vi "2D array remove invalid numbers.vi"(0 "iteration number\n(when interpolate)":i32, 1 "interpolate":bool, 2 "transpose":bool, 4 "all columns":bool=TRUE, 5 "invalid numbers list":dbl[](array[numeric])=[inf, -inf, 0.0], 6 "min":dbl=-inf, 7 "max":dbl=inf, 8 "menu":T1(ring), 9 "selected coulumn":i32, 10 "array in":dbl[][](array[numeric])=[[2.9e-06, 1031.066], [0.3000111, 1030.889], [0.6000026, 1030.51], [0.9000013, 1029.772], [1.199967, 1028.994], [1.499969, 1028.095], [1.7999, 1027.132], [2.099874, 1026.203], [2.399872, 1025.28], [2.699817, 1024.361], [2.999824, 1023.485], [3.299903, 1022.622], [3.599948, 1021.759], [3.899851, 1020.978], [4.199977, 1020.139], [4.499946, 1019.425], [4.799844, 1018.635], [5.099932, 1017.888], [5.400068, 1017.252], [5.699985, 1016.525], [5.99992, 1015.822], [6.299928, 1015.166], [6.600165, 1014.52], [6.900076, 1013.781], [7.200036, 1013.158], [7.500067, 1012.494], [7.800045, 1011.846], [8.099933, 1011.217], [8.400136, 1010.525], [8.699943, 1009.959], [9.000045, 1009.171], [9.000007, 1009.165], [0.0, 0.0], [0.0, 0.0], [0.0, 0.0], [0.0, 0.0], [0.0, 0.0], [0.0, 0.0], [0.0, 0.0], [0.0, 0.0], [0.0, 0.0], [0.0, 0.0], [0.0, 0.0], [0.0, 0.0], [0.0, 0.0], [0.0, 0.0]]) -> (3 "array out":dbl[][](array[numeric])=[[2.9e-06, 1031.066], [0.3000111, 1030.889], [0.6000026, 1030.51], [0.9000013, 1029.772], [1.199967, 1028.994], [1.499969, 1028.095], [1.7999, 1027.132], [2.099874, 1026.203], [2.399872, 1025.28], [2.699817, 1024.361], [2.999824, 1023.485], [3.299903, 1022.622], [3.599948, 1021.759], [3.899851, 1020.978], [4.199977, 1020.139], [4.499946, 1019.425], [4.799844, 1018.635], [5.099932, 1017.888], [5.400068, 1017.252], [5.699985, 1016.525], [5.99992, 1015.822], [6.299928, 1015.166], [6.600165, 1014.52], [6.900076, 1013.781], [7.200036, 1013.158], [7.500067, 1012.494], [7.800045, 1011.846], [8.099933, 1011.217], [8.400136, 1010.525], [8.699943, 1009.959], [9.000045, 1009.171], [9.000007, 1009.165], [0.0, 0.0], [0.0, 0.0], [0.0, 0.0], [0.0, 0.0], [0.0, 0.0], [0.0, 0.0], [0.0, 0.0], [0.0, 0.0], [0.0, 0.0], [0.0, 0.0], [0.0, 0.0], [0.0, 0.0], [0.0, 0.0], [0.0, 0.0]])   [LabVIEW 2025]
panel:
  # "NaN: not a number"
  # "Filter out the numbers (3 modes) for the whole or slected columns. The filtered numbers\nare removed or replaced by (sinlge or multiple times) interpolated numbers. \nWhen the numbers are to removed the rows containing the numbers are removed too.  \n\n1. Remove numbers in the list and NaN\n2. Remove numbers in the boundary\n3. Remove numbers out of the boundary\n\nFor modes 2 and 3, the default \"min\" and \"max\" numbers are -Inf and +Inf, respectively.\nIf those numbers are not wired, the operation will be done accordingly."
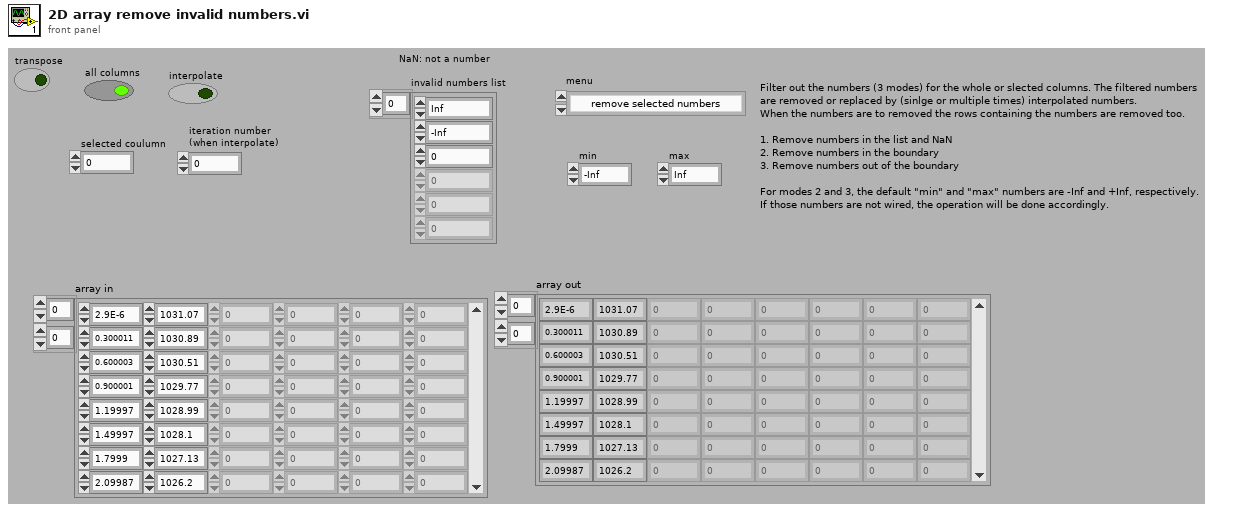
[diagram p1: front panel]
types:
  T1 = enum16{"remove selected numbers", "remove numbers within the range", "remove number out of the range", "no filtering"}
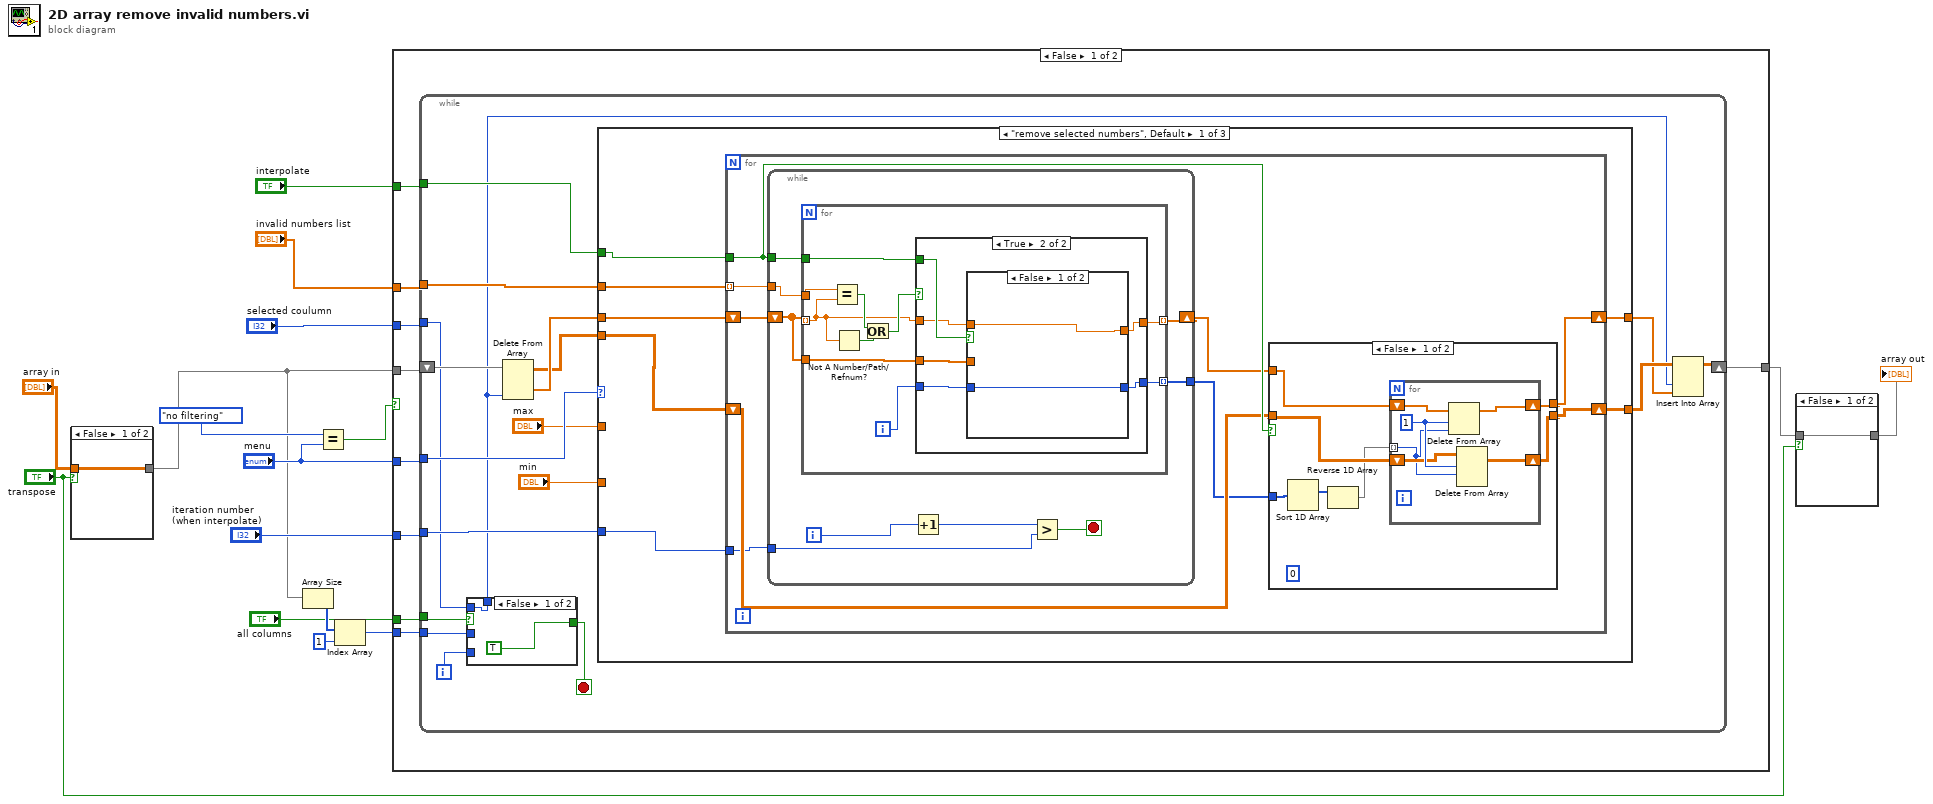
[diagram p0: block diagram]
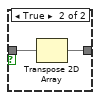
[diagram p2: hidden frame]
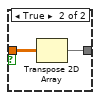
[diagram p3: hidden frame]
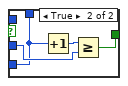
[diagram p4: hidden frame]
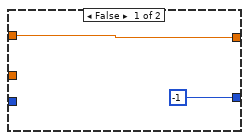
[diagram p5: hidden frame]
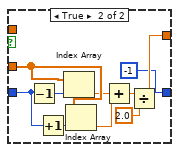
[diagram p6: hidden frame]
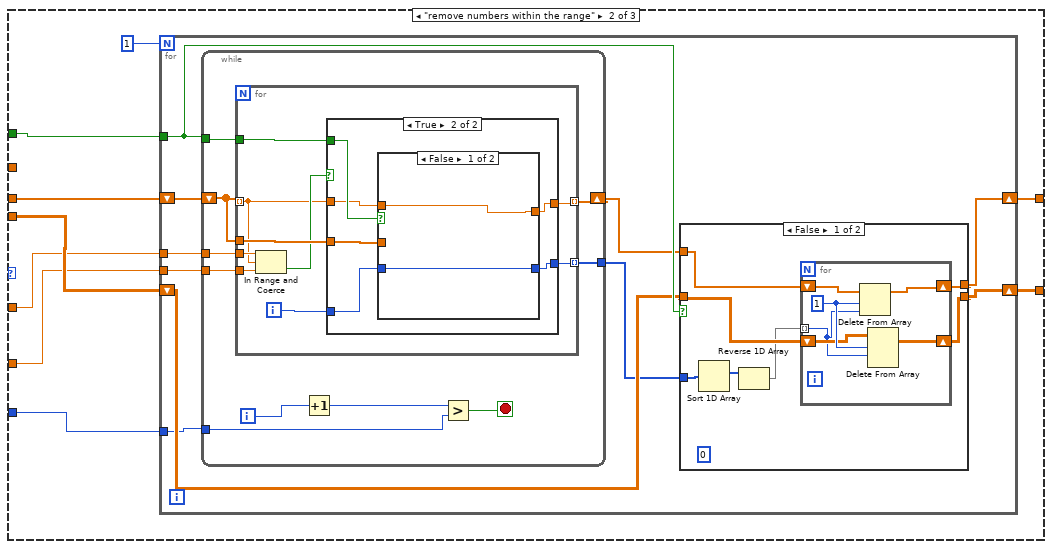
[diagram p8: hidden frame]
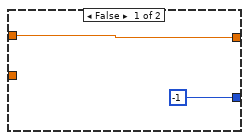
[diagram p9: hidden frame]
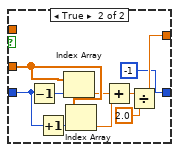
[diagram p10: hidden frame]
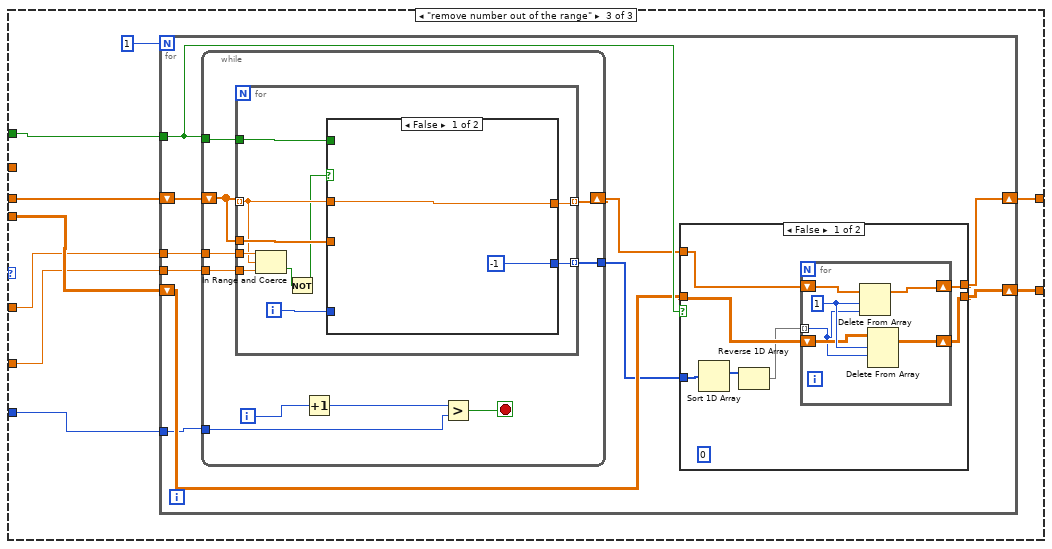
[diagram p12: hidden frame]
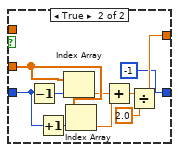
[diagram p14: hidden frame]
diagram:
  n1 = case shown="False" "transpose" {
    tunnel: "array in" -> [w17 w19]
    tunnel: [w17 w18] -> w4
    frame False {
    }
    frame True {
      n2 = Transpose 2D Array(2D array=w19) -> (transposed array=w18:dbl[][])
    }
  }
  n3 = Array Size(array=w4) -> (size(s)=w12:i32[])
  n4 = Equal?(x=T1."no filtering" ("menu"), y="menu") -> (x = y?=w7:bool)
  n5 = Index Array(array=w12, index=1) -> (element=w11:i32)
  n6 = case shown="False" w7 {
    tunnel: "interpolate" -> [w28 _]
    tunnel: "iteration number\n(when interpolate)" -> [w27 _]
    tunnel: "invalid numbers list" -> [w26 _]
    tunnel: "menu" -> [w25 _]
    tunnel: "selected coulumn" -> [w24 _]
    tunnel: w4 -> [w23 w270]
    tunnel: w11 -> [w22 _]
    tunnel: "all columns" -> [w21 _]
    tunnel: [w20 w270] -> w3
    frame False {
      n7 = while {
        tunnel: w28 -> [w46]
        tunnel: w27 -> [w42]
        tunnel: w25 -> [w40]
        shift-right: [w31] -> w20
        shift-left: w23 -> [w45]
        tunnel: w24 -> [w38]
        tunnel: w22 -> [w36]
        tunnel: w21 -> [w35]
        tunnel: w26 -> [w41]
        i -> [w37]
        stop <- w39 stop-if-true
        n8 = case shown="False" w35 {
          tunnel: [TRUE w49] -> w39
          tunnel: [w47 w51] -> w32
          tunnel: w38 -> [w47 _]
          tunnel: w37 -> [_ w51]
          tunnel: w36 -> [_ w52]
          frame False {
          }
          frame True {
            n9 = Increment(x=w51) -> (x+1=w50:i32)
            n10 = Greater Or Equal?(x=w50, y=w52) -> (x >= y?=w49:bool)
          }
        }
        n11 = Delete From Array(array=w45, index (col)=w32) -> (deleted portion=w44:dbl[], array with subset deleted=w43:dbl[][])  [unwired: 2 in]
        n12 = case shown="\"remove selected numbers\", Default" w40 {
          tunnel: w44 -> [w59 w131 w204]
          tunnel: w46 -> [w58 w130 w203]
          tunnel: [w57 w129 w202] -> w34
          tunnel: [w56 w128 w201] -> w33
          tunnel: w43 -> [w55 w127 w200]
          tunnel: w42 -> [w54 w126 w199]
          tunnel: w41 -> [w53 _ _]
          tunnel: "max" -> [_ w125 w198]
          tunnel: "min" -> [_ w124 w197]
          frame "remove selected numbers", Default {
            n13 = for {
              tunnel: w58 -> [w67]
              tunnel: w54 -> [w62]
              shift-right: [w64] -> w56
              shift-left: w59 -> [w68]
              shift-right: [w65] -> w57
              shift-left: w55 -> [w63]
              tunnel: w53 -> [w60] mode=indexing
              n14 = while {
                shift-right: [w76] -> w66
                shift-left: w68 -> [w77]
                tunnel: w67 -> [w72]
                tunnel: [w71] -> w61
                tunnel: w62 -> [w70]
                tunnel: w60 -> [w69]
                i -> [w75]
                stop <- w74 stop-if-true
                n15 = for {
                  tunnel: w77 -> [w86]
                  tunnel: w72 -> [w84]
                  tunnel: [w83] -> w71 mode=indexing
                  tunnel: w77 -> [w78] mode=indexing
                  tunnel: [w87] -> w76 mode=indexing
                  tunnel: w69 -> [w81]
                  i -> [w85]
                  n16 = Equal?(x=w81, y=w78) -> (x = y?=w82:bool)
                  n17 = Not A Number/Path/Refnum?(number/path/refnum=w78) -> (NaN/Path/Refnum?=w80:bool)
                  n18 = Or(x=w82, y=w80) -> (x .or. y?=w79:bool)
                  n19 = case shown="True" w79 {
                    tunnel: [w89 w90] -> w87
                    tunnel: w78 -> [w89 w91]
                    tunnel: w86 -> [_ w95]
                    tunnel: w85 -> [_ w94]
                    tunnel: w84 -> [_ w93]
                    tunnel: [-1 w92] -> w83
                    frame False {
                    }
                    frame True {
                      n20 = case shown="False" w93 {
                        tunnel: w95 -> [_ w107]
                        tunnel: w94 -> [w97 w106]
                        tunnel: [w96 w99] -> w90
                        tunnel: [w97 -1] -> w92
                        tunnel: w91 -> [w96 _]
                        frame False {
                        }
                        frame True {
                          n21 = Decrement(x=w106) -> (x-1=w105:i32)
                          n22 = Increment(x=w106) -> (x+1=w104:i32)
                          n23 = Index Array(array=w107, index=w105) -> (element=w103:dbl)
                          n24 = Index Array(array=w107, index=w104) -> (element=w102:dbl)
                          n25 = Add(x=w103, y=w102) -> (x+y=w101:dbl)
                          n26 = Divide(x=w101, y=2.0) -> (x/y=w99:dbl)
                        }
                      }
                    }
                  }
                }
                n27 = Increment(x=w75) -> (x+1=w73:i32)
                n28 = Greater?(x=w73, y=w70) -> (0:w74:bool)
              }
              n29 = case shown="False" w67 {
                tunnel: [w113 w122] -> w64
                tunnel: w66 -> [w111 w122]
                tunnel: [w112 w121] -> w65
                tunnel: w63 -> [w114 w121]
                tunnel: w61 -> [w108 _]
                frame False {
                  (unwired) 0
                  n30 = Sort 1D Array(array=w108) -> (sorted array=w110:i32[])
                  n31 = Reverse 1D Array(array=w110) -> (reversed array=w109:i32[])
                  n32 = for {
                    tunnel: w109 -> [w115] mode=indexing
                    shift-right: [w118] -> w113
                    shift-left: w111 -> [w120]
                    shift-right: [w116] -> w112
                    shift-left: w114 -> [w117]
                    w119 = 1 ("length")
                    n33 = Delete From Array(array=w120, length=w119, index=w115) -> (array with subset deleted=w118:dbl[])  [unwired: 1 out]
                    n34 = Delete From Array(array=w117, length=w119, index (row)=w115) -> (array with subset deleted=w116:dbl[][])  [unwired: 1 in, 1 out]
                  }
                }
                frame True {
                }
              }
            }
          }
          frame "remove numbers within the range" {
            n35 = for {
              N: 1 -> [_]
              tunnel: w130 -> [w140]
              tunnel: w126 -> [w135]
              shift-right: [w137] -> w128
              shift-left: w131 -> [w141]
              shift-right: [w138] -> w129
              shift-left: w127 -> [w136]
              tunnel: w125 -> [w133]
              tunnel: w124 -> [w132]
              n36 = while {
                shift-right: [w150] -> w139
                shift-left: w141 -> [w151]
                tunnel: w140 -> [w146]
                tunnel: [w145] -> w134
                tunnel: w135 -> [w144]
                tunnel: w133 -> [w143]
                tunnel: w132 -> [w142]
                i -> [w149]
                stop <- w148 stop-if-true
                n37 = for {
                  tunnel: w151 -> [w159]
                  tunnel: w146 -> [w157]
                  tunnel: [w156] -> w145 mode=indexing
                  tunnel: w151 -> [w152] mode=indexing
                  tunnel: [w160] -> w150 mode=indexing
                  tunnel: w143 -> [w155]
                  tunnel: w142 -> [w154]
                  i -> [w158]
                  n38 = In Range and Coerce(upper limit=w155, x=w152, lower limit=w154) -> (In Range?=w153:bool)  [unwired: 1 out]
                  n39 = case shown="True" w153 {
                    tunnel: [w162 w163] -> w160
                    tunnel: w152 -> [w162 w164]
                    tunnel: w159 -> [_ w168]
                    tunnel: w158 -> [_ w167]
                    tunnel: w157 -> [_ w166]
                    tunnel: [-1 w165] -> w156
                    frame False {
                    }
                    frame True {
                      n40 = case shown="False" w166 {
                        tunnel: w168 -> [_ w180]
                        tunnel: w167 -> [w170 w179]
                        tunnel: [w169 w172] -> w163
                        tunnel: [w170 -1] -> w165
                        tunnel: w164 -> [w169 _]
                        frame False {
                        }
                        frame True {
                          n41 = Decrement(x=w179) -> (x-1=w178:i32)
                          n42 = Increment(x=w179) -> (x+1=w177:i32)
                          n43 = Index Array(array=w180, index=w178) -> (element=w176:dbl)
                          n44 = Index Array(array=w180, index=w177) -> (element=w175:dbl)
                          n45 = Add(x=w176, y=w175) -> (x+y=w174:dbl)
                          n46 = Divide(x=w174, y=2.0) -> (x/y=w172:dbl)
                        }
                      }
                    }
                  }
                }
                n47 = Increment(x=w149) -> (x+1=w147:i32)
                n48 = Greater?(x=w147, y=w144) -> (0:w148:bool)
              }
              n49 = case shown="False" w140 {
                tunnel: [w186 w195] -> w137
                tunnel: w139 -> [w184 w195]
                tunnel: [w185 w194] -> w138
                tunnel: w136 -> [w187 w194]
                tunnel: w134 -> [w181 _]
                frame False {
                  (unwired) 0
                  n50 = Sort 1D Array(array=w181) -> (sorted array=w183:i32[])
                  n51 = Reverse 1D Array(array=w183) -> (reversed array=w182:i32[])
                  n52 = for {
                    tunnel: w182 -> [w188] mode=indexing
                    shift-right: [w191] -> w186
                    shift-left: w184 -> [w193]
                    shift-right: [w189] -> w185
                    shift-left: w187 -> [w190]
                    w192 = 1 ("length")
                    n53 = Delete From Array(array=w193, length=w192, index=w188) -> (array with subset deleted=w191:dbl[])  [unwired: 1 out]
                    n54 = Delete From Array(array=w190, length=w192, index (row)=w188) -> (array with subset deleted=w189:dbl[][])  [unwired: 1 in, 1 out]
                  }
                }
                frame True {
                }
              }
            }
          }
          frame "remove number out of the range" {
            n55 = for {
              N: 1 -> [_]
              tunnel: w203 -> [w213]
              tunnel: w199 -> [w208]
              shift-right: [w210] -> w201
              shift-left: w204 -> [w214]
              shift-right: [w211] -> w202
              shift-left: w200 -> [w209]
              tunnel: w198 -> [w206]
              tunnel: w197 -> [w205]
              n56 = while {
                shift-right: [w223] -> w212
                shift-left: w214 -> [w224]
                tunnel: w213 -> [w219]
                tunnel: [w218] -> w207
                tunnel: w208 -> [w217]
                tunnel: w206 -> [w216]
                tunnel: w205 -> [w215]
                i -> [w222]
                stop <- w221 stop-if-true
                n57 = for {
                  tunnel: w224 -> [w233]
                  tunnel: w219 -> [w231]
                  tunnel: [w230] -> w218 mode=indexing
                  tunnel: w224 -> [w227] mode=indexing
                  tunnel: [w234] -> w223 mode=indexing
                  tunnel: w216 -> [w229]
                  tunnel: w215 -> [w228]
                  i -> [w232]
                  n58 = In Range and Coerce(upper limit=w229, x=w227, lower limit=w228) -> (In Range?=w226:bool)  [unwired: 1 out]
                  n59 = Not(x=w226) -> (.not. x?=w225:bool)
                  n60 = case shown="False" w225 {
                    tunnel: [w236 w237] -> w234
                    tunnel: w227 -> [w236 w238]
                    tunnel: w233 -> [_ w242]
                    tunnel: w232 -> [_ w241]
                    tunnel: w231 -> [_ w240]
                    tunnel: [-1 w239] -> w230
                    frame False {
                    }
                    frame True {
                      n61 = case shown="False" w240 {
                        tunnel: w242 -> [_ w254]
                        tunnel: w241 -> [w244 w253]
                        tunnel: [w243 w246] -> w237
                        tunnel: [w244 -1] -> w239
                        tunnel: w238 -> [w243 _]
                        frame False {
                        }
                        frame True {
                          n62 = Decrement(x=w253) -> (x-1=w252:i32)
                          n63 = Increment(x=w253) -> (x+1=w251:i32)
                          n64 = Index Array(array=w254, index=w252) -> (element=w250:dbl)
                          n65 = Index Array(array=w254, index=w251) -> (element=w249:dbl)
                          n66 = Add(x=w250, y=w249) -> (x+y=w248:dbl)
                          n67 = Divide(x=w248, y=2.0) -> (x/y=w246:dbl)
                        }
                      }
                    }
                  }
                }
                n68 = Increment(x=w222) -> (x+1=w220:i32)
                n69 = Greater?(x=w220, y=w217) -> (0:w221:bool)
              }
              n70 = case shown="False" w213 {
                tunnel: [w260 w269] -> w210
                tunnel: w212 -> [w258 w269]
                tunnel: [w259 w268] -> w211
                tunnel: w209 -> [w261 w268]
                tunnel: w207 -> [w255 _]
                frame False {
                  (unwired) 0
                  n71 = Sort 1D Array(array=w255) -> (sorted array=w257:i32[])
                  n72 = Reverse 1D Array(array=w257) -> (reversed array=w256:i32[])
                  n73 = for {
                    tunnel: w256 -> [w262] mode=indexing
                    shift-right: [w265] -> w260
                    shift-left: w258 -> [w267]
                    shift-right: [w263] -> w259
                    shift-left: w261 -> [w264]
                    w266 = 1 ("length")
                    n74 = Delete From Array(array=w267, length=w266, index=w262) -> (array with subset deleted=w265:dbl[])  [unwired: 1 out]
                    n75 = Delete From Array(array=w264, length=w266, index (row)=w262) -> (array with subset deleted=w263:dbl[][])  [unwired: 1 in, 1 out]
                  }
                }
                frame True {
                }
              }
            }
          }
        }
        n76 = Insert Into Array(array=w34, index (col)=w32, new element=w33) -> (w31:dbl[][])  [unwired: 1 in]
      }
    }
    frame True {
    }
  }
  n77 = case shown="False" "transpose" {
    tunnel: w3 -> [w271 w273]
    tunnel: [w271 w272] -> w2
    frame False {
    }
    frame True {
      n78 = Transpose 2D Array(2D array=w273) -> (transposed array=w272:dbl[][])
    }
  }
  "array out" <- w2
